vi "Set enPassant flag.vi"(8 "error in (no error)":errorcluster, 10 "enPassant target":T1={"File"=enum."d", "Rank"=enum."4"}, 11 "Position in":refnum<class "Position.lvclass">) -> (0 "error out":errorcluster, 3 "Position out":refnum<class "Position.lvclass">)   [LabVIEW 2016, in "Chesslib.lvlib" / "Position.lvclass"]
uses:
  Position.lvclass
  typedef/Square.ctl
  typedef/File.ctl
  typedef/Rank.ctl
  Position.lvclass/Position.ctl
  Chesslib.lvlib
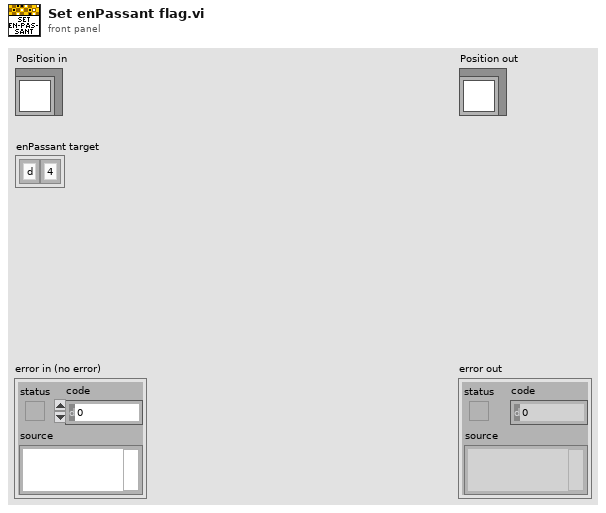
[diagram p1: front panel]
types:
  T1 = typedef "Chesslib.lvlib/Square.ctl" = cluster{"File":T2, "Rank":T3}
  T2 = typedef "Chesslib.lvlib/File.ctl" = enum8{"a", "b", "c", "d", "e", "f", "g", "h"}
  T3 = typedef "Chesslib.lvlib/Rank.ctl" = enum8{"1", "2", "3", "4", "5", "6", "7", "8"}
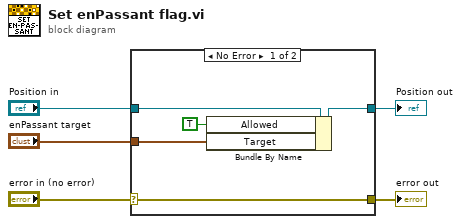
[diagram p0: block diagram]
diagram:
  n1 = case shown="No Error" "error in (no error)" {
    selector: "error in (no error)" -> [w9 w12]
    tunnel: [w9 w12] -> w4
    tunnel: [w8 w11] -> w2
    tunnel: "Position in" -> [w10 w11]
    tunnel: "enPassant target" -> [w6 _]
    frame No Error {
      n2 = Bundle By Name(cluster=w10, "Allowed"=TRUE ("en Passant.Allowed"), "Target"=w6) -> (w8:refnum<class "Position.lvclass">)
    }
    frame Error {
    }
  }
  "error out" <- w4
  "Position out" <- w2
